vi "Get In Range Trigger.vi"(7 "Trigger Direction":T2, 8 "error in (no error)":errorcluster, 11 "Item Ref in":T3 format="%.0x") -> (0 "error out":errorcluster, 2 "In Range Trigger":T1, 3 "Item Ref out":T3 format="%.0x")   [LabVIEW 2015, in "Waveform Data Logger Shared.lvlib"]
uses:
  Waveform Data Logger Shared.lvlib
  <vilib>/NI Veristand/Custom Device API/Custom Device Item Ref.ctl
  Types/Trigger Direction.ctl
  Types/In Range Trigger.ctl
  Globals/Property Strings.vi
  <vilib>/NI Veristand/Custom Device API/Get Item Property (Double).vi
  <vilib>/NI Veristand/Custom Device API/Get Item Property (Boolean).vi
  <vilib>/NI VeriStand/Custom Device API/Custom Device API.lvlib
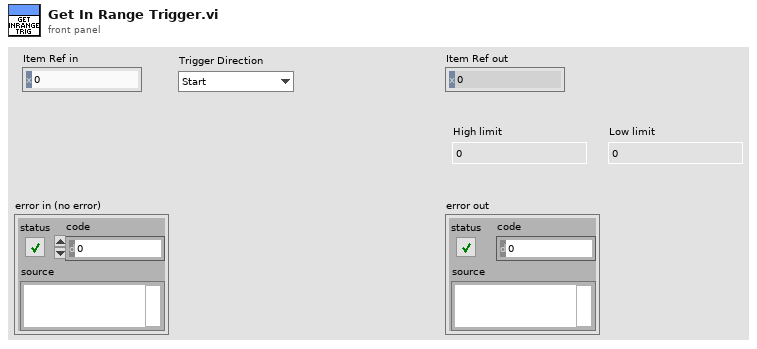
[diagram p1: front panel]
types:
  T1 = typedef "Waveform Data Logger Shared.lvlib/In Range Trigger.ctl" = cluster{"High limit":dbl, "Low limit":dbl, "Invert?":bool}
  T2 = typedef "Waveform Data Logger Shared.lvlib/Trigger Direction.ctl" = enum16{"Start", "Stop"}
  T3 = typedef "Custom Device API.lvlib/Custom Device Item Ref.ctl" = u64
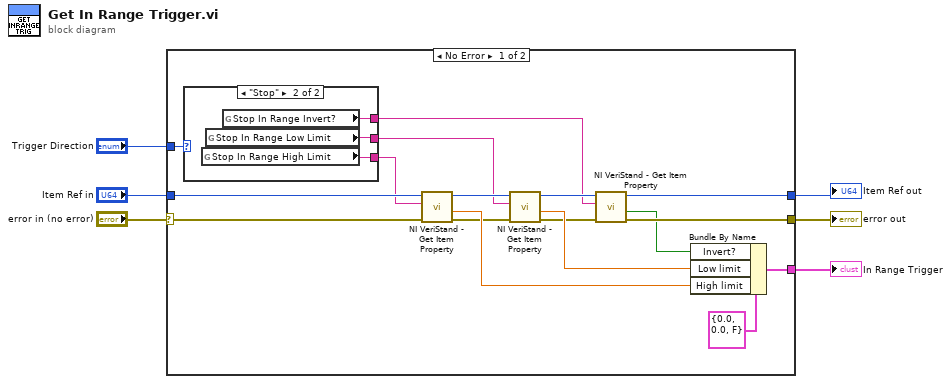
[diagram p0: block diagram]
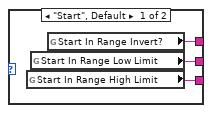
[diagram p2: hidden frame]
diagram:
  n1 = case shown="No Error" "error in (no error)" {
    selector: "error in (no error)" -> [w21 w30]
    tunnel: [w10 w31] -> w6
    tunnel: [w12 w30] -> w5
    tunnel: "Item Ref in" -> [w20 w31]
    tunnel: "Trigger Direction" -> [w23 _]
    tunnel: [w7 _] -> w1
    frame No Error {
      n2 = case shown="\"Stop\"" w23 {
        tunnel: [w26 w28] -> w15
        tunnel: [w25 w27] -> w19
        tunnel: [w24 w29] -> w9
        frame "Start", Default {
          n3 = global read "Property Strings.vi" "Start In Range High Limit"() -> (w25:string)
          n4 = global read "Property Strings.vi" "Start In Range Low Limit"() -> (w26:string)
          n5 = global read "Property Strings.vi" "Start In Range Invert?"() -> (w24:string)
        }
        frame "Stop" {
          n6 = global read "Property Strings.vi" "Stop In Range High Limit"() -> (w27:string)
          n7 = global read "Property Strings.vi" "Stop In Range Low Limit"() -> (w28:string)
          n8 = global read "Property Strings.vi" "Stop In Range Invert?"() -> (w29:string)
        }
      }
      n9 = call-poly <vilib>:"NI VeriStand - Get Item Property.vi"("error in (no error)"=w21, "Property Name"=w19, "Item Ref in"=w20) -> ("error out"=w17:errorcluster, "Value"=w18:dbl, "Item Ref out"=w16:T3)  [unwired: 1 in, 5 out]
      n10 = call-poly <vilib>:"NI VeriStand - Get Item Property.vi"("error in (no error)"=w17, "Property Name"=w15, "Item Ref in"=w16) -> ("error out"=w13:errorcluster, "Value"=w14:dbl, "Item Ref out"=w11:T3)  [unwired: 1 in, 5 out]
      n11 = call-poly <vilib>:"NI VeriStand - Get Item Property.vi"("error in (no error)"=w13, "Property Name"=w9, "Item Ref in"=w11) -> ("error out"=w12:errorcluster, "Value"=w8:bool, "Item Ref out"=w10:T3)  [unwired: 1 in, 5 out]
      n12 = Bundle By Name(cluster=T1 {"High limit"=0.0, "Low limit"=0.0, "Invert?"=FALSE} ("In Range Trigger"), "Invert?"=w8, "Low limit"=w14, "High limit"=w18) -> (w7:T1)
    }
    frame Error {
    }
  }
  "Item Ref out" <- w6
  "error out" <- w5
  "In Range Trigger" <- w1
